vi "codigo 2.vi"() -> ()   [LabVIEW 2019]
panel:
  out "Waveform Chart":dbl(graph)
  in  "Slide":dbl(slide) scale=0.0..10.0
  out "Numeric 2":dbl
  in  "Numeric":dbl
  in  "Cancel Button":bool
  in  "OK Button":bool
  in  "stop":bool
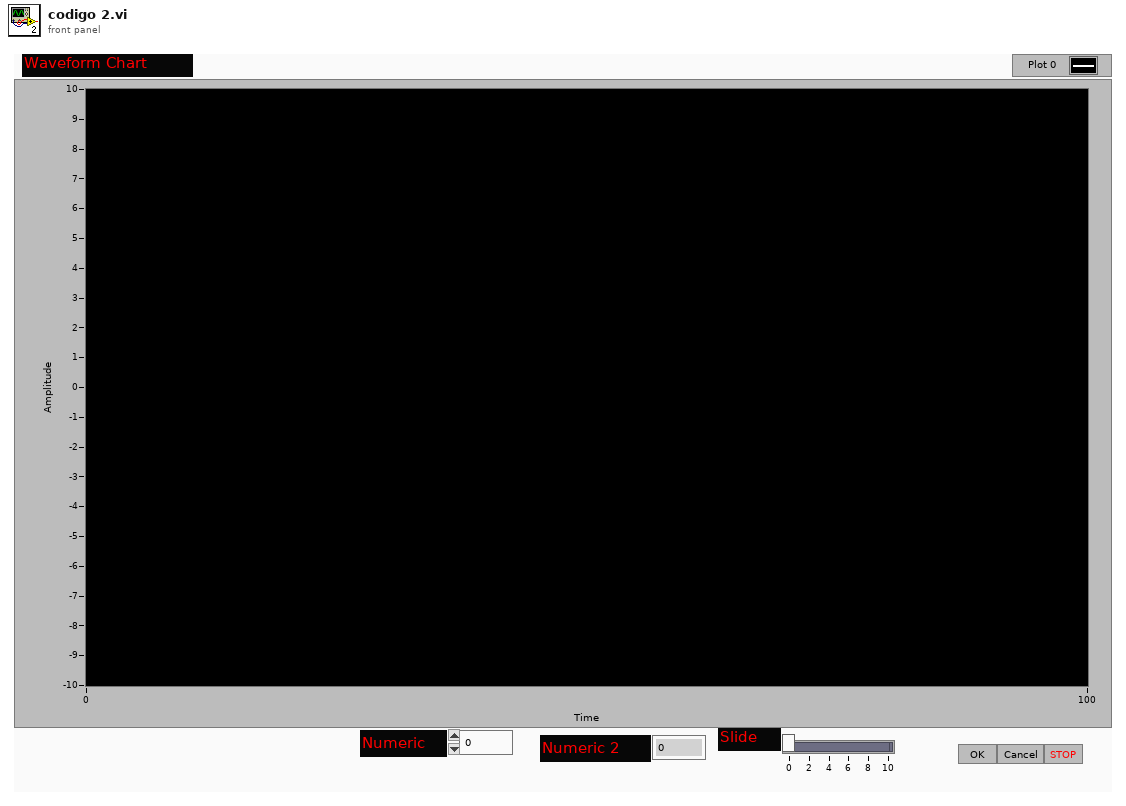
[diagram p1: front panel]
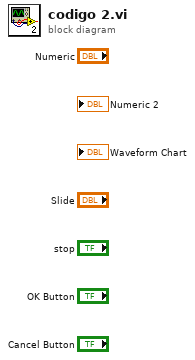
[diagram p0: block diagram]
diagram:
